vi "Calculate time.vi"(11 "Status":T1 {"Setting"."X Pos." scale=-2.0..2.0; "Setting"."Y Pos." scale=-2.0..2.0}) -> (3 "数值":dbl)   [LabVIEW 2013]
uses:
  init & communication/init-status.ctl
  init & communication/Setting.ctl
  init & communication/event-package.ctl
  init & communication/Event1.ctl
  init & communication/data-package.ctl
  init & communication/Event.ctl
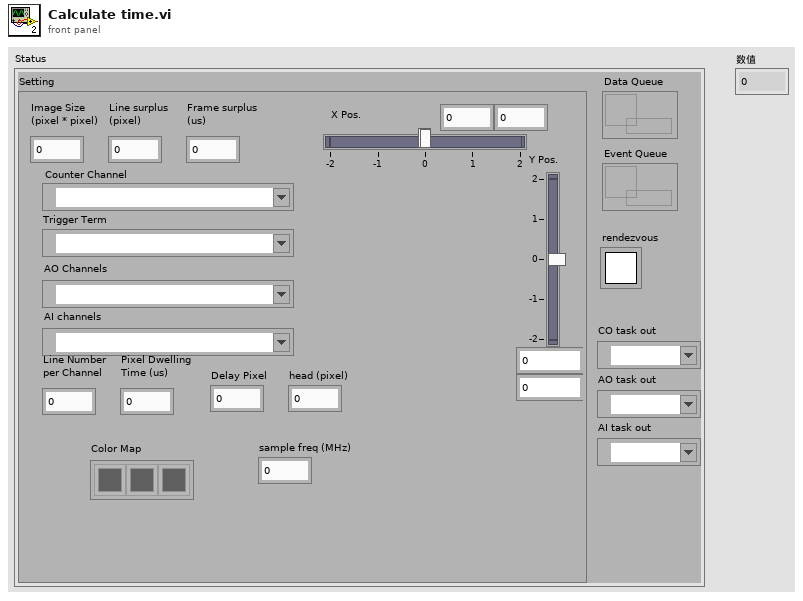
[diagram p1: front panel]
types:
  T1 = typedef "init-status.ctl" = cluster{"Setting":T2, "Event Queue":refnum<queue>, "Data Queue":refnum<queue>, "rendezvous":T3, "CO task out":refnum<k21>, "AO task out":refnum<k21>, "AI task out":refnum<k21>}
  T2 = typedef "Setting.ctl" = cluster{"Image Size\n(pixel * pixel)":i32, "Counter Channel":tag, "Trigger Term":tag, "AO Channels":tag, "Y Pos.":cluster{dbl, dbl}, "X Pos.":cluster{dbl, dbl}, "Line surplus\n(pixel)":i32, "Frame surplus\n(us)":i32, "AI channels":tag, "Line Number\nper Channel":i32, "Delay Pixel":i32, "Pixel Dwelling\nTime (us)":i32, "Color Map":u32[], "head (pixel)":i32, "sample freq (MHz)":dbl}
  T3 = typedef "Rendezvous RefNum" = refnum<k1>
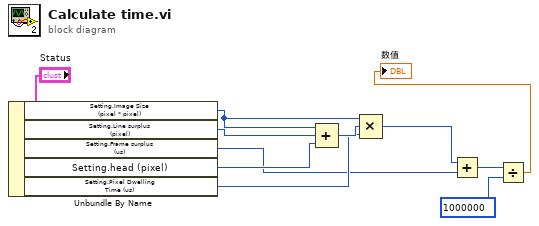
[diagram p0: block diagram]
diagram:
  n1 = Unbundle By Name("Status") -> ("Setting.Image Size\n(pixel * pixel)"=w7:i32, "Setting.Line surplus\n(pixel)"=w10:i32, "Setting.Frame surplus\n(us)"=w4:i32, "Setting.head (pixel)"=w9:i32, "Setting.Pixel Dwelling\nTime (us)"=w6:i32)
  n2 = Compound Arithmetic op=ADD(w7, w10, w9) -> (w8:i32)
  n3 = Compound Arithmetic op=MULTIPLY(w7, w8, w6) -> (w5:i32)
  n4 = Add(x=w5, y=w4) -> (x+y=w3:i32)
  n5 = Divide(x=w3, y=1000000) -> (x/y=→"数值":dbl)
